vi "FA_ConvertToSharedVariables.vi"(8 "Error In":errorcluster, 11 "Config":T1) -> (0 "Error Out":errorcluster, 3 "SV":T3)   [LabVIEW 2014, in "FA_SharedVariables.lvlib"]
doc: "Converts from the general config typedef to a shared variable typedef"
uses:
  FA_SharedVariables.lvlib
  FA_SharedVariables.ctl
  FA_NativeTypes API/source/VI Source/FA_Config.ctl
  FA_LocalStore API/source/VI Source/FA_LSSpecialTypes.ctl
  FA_LocalStore API/source/VI Source/FA_LocalStore.lvlib
  FA_NativeTypes API/source/VI Source/FA_NativeTypes.lvlib
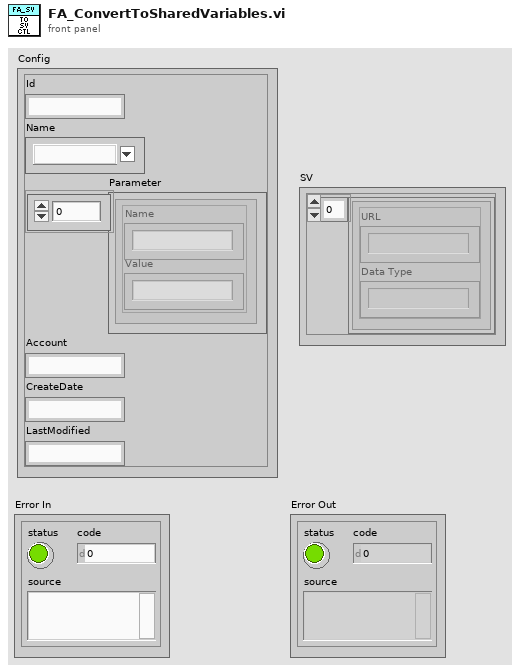
[diagram p1: front panel]
types:
  T1 = typedef "FA_NativeTypes.lvlib/FA_Config.ctl" = cluster{"Id":string, "Name":T2, "Parameter":cluster{"Name":string, "Value":string}[], "Account":string, "CreateDate":string, "LastModified":string}
  T2 = typedef "FA_LocalStore.lvlib/FA_LSSpecialTypes.ctl" = string
  T3 = typedef "FA_SharedVariables.lvlib/FA_SharedVariables.ctl" = cluster{"Shared Variables":cluster{"URL":string, "Data Type":string}[]}
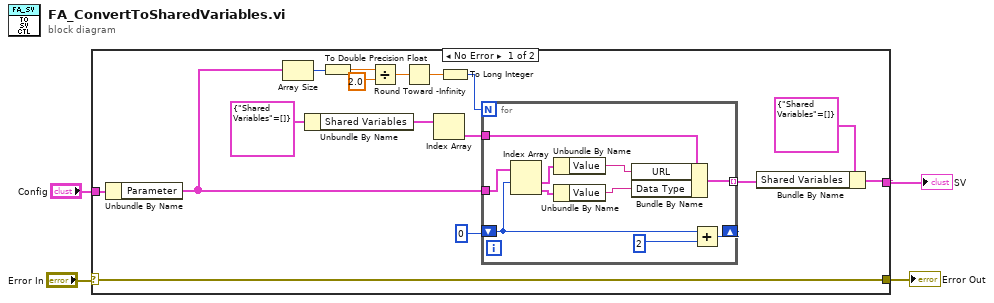
[diagram p0: block diagram]
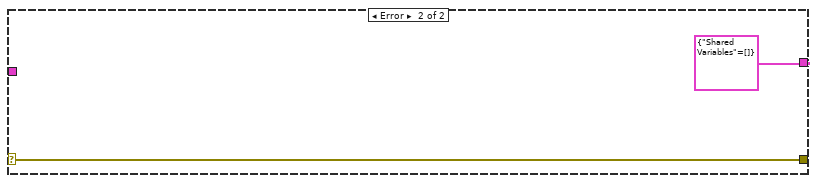
[diagram p2: hidden frame]
diagram:
  n1 = case shown="No Error" "Error In" {
    selector: "Error In" -> [w10 w32]
    tunnel: "Config" -> [w20 _]
    tunnel: [w10 w32] -> w2
    tunnel: [w5 T3 {"Shared Variables"=[]} ("Shared Variable")] -> w1
    frame No Error {
      n2 = Unbundle By Name(w20) -> ("Parameter"=w11:cluster{"Name":string, "Value":string}[])
      n3 = Array Size(array=w11) -> (size(s)=w17:i32)
      n4 = Unbundle By Name(T3 {"Shared Variables"=[]} ("Shared Variable")) -> ("Shared Variables"=w8:cluster{"URL":string, "Data Type":string}[])
      n5 = To Double Precision Float(number=w17) -> (double precision float=w16:dbl)
      n6 = Divide(x=w16, y=2.0) -> (x/y=w14:dbl)
      n7 = Round Toward -Infinity(1:w14) -> (0:w12:dbl)
      n8 = Index Array(array=w8) -> (element=w18:cluster{"URL":string, "Data Type":string})  [unwired: 1 in]
      n9 = To Long Integer(number=w12) -> (32bit integer=w13:i32)
      n10 = for {
        N: w13 -> [_]
        tunnel: w11 -> [w30]
        shift-right: [w27] -> _
        shift-left: 0 ("index") -> [w29]
        tunnel: w18 -> [w25]
        tunnel: [w24] -> w6 mode=indexing
        n11 = Index Array(array=w30, index #1=w29) -> (element #1=w22:cluster{"Name":string, "Value":string}, element #2=w21:cluster{"Name":string, "Value":string})  [unwired: 1 in]
        n12 = Unbundle By Name(w22) -> ("Value"=w26:string)
        n13 = Unbundle By Name(w21) -> ("Value"=w23:string)
        n14 = Bundle By Name(cluster=w25, "URL"=w26, "Data Type"=w23) -> (w24:cluster{"URL":string, "Data Type":string})
        n15 = Add(x=w29, y=2) -> (x+y=w27:i32)
      }
      n16 = Bundle By Name(cluster=T3 {"Shared Variables"=[]} ("Shared Variable"), "Shared Variables"=w6) -> (w5:T3)
    }
    frame Error {
    }
  }
  "Error Out" <- w2
  "SV" <- w1
